vi "获取变量名称.vi"(1 "属性数组":T1(array[cluster])) -> (0 "名称数组":string[](array[string]))   [LabVIEW 2014]
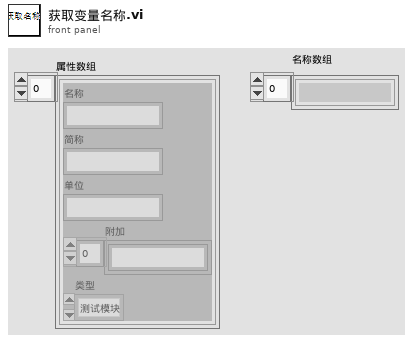
[diagram p1: front panel]
types:
  T1 = cluster{"名称":string, "简称":string, "单位":string, "附加":string[], "类型":enum16{"测试模块", "FPGA", "cRIO", "其他设备", "总体展示"}}[]
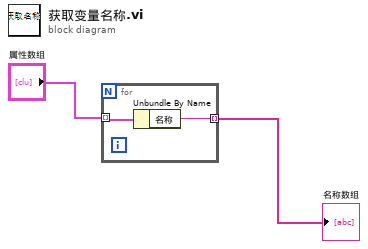
[diagram p0: block diagram]
diagram:
  n1 = for {
    tunnel: "属性数组" -> [w4] mode=indexing
    tunnel: [w3] -> w2 mode=indexing
    n2 = Unbundle By Name(w4) -> ("名称"=w3:string)
  }
  "名称数组" <- w2
